vi "Complete Algorithm_Host.vi"() -> ()   [LabVIEW 2011]
uses:
  <vilib>/measure/NI_MAPro.lvlib
  <vilib>/Analysis/NI_AALBase.lvlib
  FFT/Controls/FFT States.ctl
  <vilib>/measure/maspectr.llb/FFT Spectrum (Mag-Phase) for 1 Chan (CDB).vi
  <vilib>/Analysis/1siggen.llb/Ramp Pattern by Samples.vi
  Interpolation Block/Controls/Interpolation Input Data.ctl
  <vilib>/Analysis/NI_AALPro.lvlib
  <vilib>/Analysis/2dsp.llb/Real FFT.vi
  <vilib>/gmath/NI_Gmath.lvlib
  FFT/Controls/FFT Parameters.ctl
panel:
  out "Resampled Waveform Error":dbl[](graph)=[-6.976252814558266, -5.323343553412211, -2.8114333153546744, -26.54772585626159, -19.783463943885028, -24.955368759801782, -31.021231527647238, -27.6461877092507, -38.95671779693381, -29.146757893293778, -40.920500463104865, -29.778667799092602, -30.651480033843615, -39.617647950762674, -29.777119057976908, -35.747085008088305, -35.2985019790654, -37.76767677188048, -33.9462465942451, -30.02327803942113, -39.37688378105776, -35.94385793381323, -35.585106057981605, -40.48040927607361, -32.74968635815885, -36.438287617816435, -47.755067442121316, -40.45338682146091, -52.23635514643328, -40.6295428448561, -38.1524909017659, -48.76110841180686, -40.71433935621975, -39.00688364486796, -56.49784789209585, -37.42986222843402, -40.49625037212847, -44.06886067307057, -38.31525964353108, -59.63457027143055, -35.566588313612634, -33.467351968403946, -36.68413625267246, -41.04536841104639, -42.31435254051097, -36.274070107607145, -37.150764121682805, -50.332950824589815, -46.20156369462504, -46.444900910375225, -44.8364219648814, -48.57917680413567, -42.19794262901505, -40.506737237586975, -52.63002253901345, -39.72758659866716, -38.214786945688516, -39.56035908067337, -43.32060173475149, -39.61076431387224, -33.093522184387204, -34.74046406069414, -45.152114353755366, -38.20642899575148, -42.09609113759559, -41.768976367924466, -38.66318028792905, -38.4756737843668, -39.924187998371096, -46.05349347381723, -35.49027459608772, -36.025415041989326, -38.51092517659433, -36.83569854602486, -40.795380624021725, -36.35991369515506, -37.81728427386544, -44.61046277229856, -35.266016721014964, -35.92322715684338, -42.88567587562287, -50.74251290714233, -44.872042376101916, -42.68123807149777, -42.92436430457484, -48.84492734632382, -45.3696804814589, -38.37702895182521, -40.36098970624832, -48.510609418962495, -57.25548500472812, -43.979468134992715, -38.14224729316644, -40.56618511041606, -58.13679214274917, -44.759022108404935, -40.256764450613, -41.685001222819444, -54.61994454936558, -44.38945314872701, -49.93473371978812, -46.25638908324654, -42.539518328159865, -45.28773309215987, -43.23721587175819, -45.564359245981514, -46.961044473626615, -41.32558704191926, -38.125744733097655]
  out "FFT_FXP_no DIT":dbl[](graph)=[-0.9553570049207104, 0.6968999494108972, 3.2074240707672486, -20.53122498149444, -13.77089446014236, -18.952463060127535, -25.022087351671377, -21.655924863873462, -32.972655817656346, -23.178155409959732, -34.96764173487915, -23.830599429203577, -24.72530525148686, -33.696009783345744, -23.883798703280526, -29.872860366292603, -29.438514987857264, -31.94494876745275, -28.134798131521784, -24.23918297363493, -33.63738541391448, -30.215293162386203, -29.890534838760058, -34.805342346114784, -27.123370304893385, -30.839734571250396, -42.17935864808424, -34.92729722281159, -46.65167705453899, -35.156781588661715, -32.71759437126826, -43.39065085727536, -35.35602088973465, -33.720145839352995, -51.22083266003117, -32.22975713342345, -35.372416231632016, -38.961220511182894, -33.295472896454925, -54.94205288567625, -30.643481005262174, -28.613588128886647, -31.89687360197505, -36.34212825746688, -37.630998520773005, -31.664986633794463, -32.60179747579538, -45.75845140392847, -41.84167849659361, -42.09857689345015, -40.617829297597325, -44.43194429667791, -38.11044261216089, -36.528827231710956, -48.782090563932016, -35.920982262632904, -34.50760172914073, -35.91963395980357, -39.7684802539758, -36.13416975134405, -29.703949311666285, -31.44846989771336, -41.95513728241616, -35.10351644257866, -39.07605566599686, -38.87160754828359, -35.91749374911157, -35.85331514008895, -37.44076426648204, -43.70958159602134, -33.21932185799169, -33.9061230773539, -36.55098574885896, -34.9837064659399, -39.08072335574801, -34.794348852725776, -36.39048296432991, -43.31555914578375, -34.19729522033075, -35.02592866181829, -42.21011656437949, -49.98820340744261, -44.37636412014499, -42.393601328796876, -42.88625468811113, -49.03715936994228, -45.71970468705827, -38.917038799967656, -41.10409295431466, -49.48714628994594, -58.85648271093962, -45.42701062252409, -39.84728347746511, -42.54601837493462, -60.621507019043705, -47.14439309014662, -42.94569780155637, -44.761084889164124, -57.83927091459509, -47.97668555883114, -54.11859137929727, -50.610961848127296, -47.29689223076528, -50.46072316096139, -48.986236804948476, -52.083879275586, -53.307091387367734, -48.16224363052139, -45.443188472860484, -45.23440881714418, -47.85854889637821, -56.27836973151929, -54.9658463374032, -52.46594288951086, -66.34887368032327, -55.304784228123715, -52.19923351123122, -49.138384495401304, -49.26606066713251, -57.96592937153396, -60.3194968415907, -55.628260569108406, -58.20499964743555, -68.60615252726132]
  in  "Resample Waveform Size":i32=1024
  out "Error 2":dbl[](graph)=[43.28680336773397, 54.874209998377815, 63.40667927216815, 43.19214378295915, 52.4550850459606, 49.22125785617935, 44.738870122314516, 49.45267259284084, 39.30177705005138, 50.134555753031705, 39.275704089007256, 51.245104293962626, 51.127749856906036, 42.85648338602506, 53.340338006756994, 47.96924132299105, 48.97797635960519, 47.034930612021746, 51.352355468446454, 55.7444416762564, 46.8358322946451, 50.69208531689444, 51.454318833795625, 46.94450536240401, 55.04425575816844, 51.709561920450575, 40.7327536810958, 48.36152013811606, 36.89368738030214, 48.80452194457727, 51.57523466078294, 41.25059427183906, 49.5722700549092, 51.54611873091486, 34.313540452847406, 53.63236777747285, 50.80970056229957, 47.47407920925422, 53.45829484965432, 32.363554263910956, 56.65036641185069, 58.962975235045974, 55.95436745637467, 51.796359091271164, 50.72587252279395, 56.960137493066384, 56.273108272838066, 43.27645317017654, 47.589411598739304, 47.523847575579595, 49.30645397147554, 45.73432415131559, 52.282815875412304, 54.1380385934558, 42.17565050739418, 55.23597705017646, 56.90376805485219, 55.710389681351565, 52.09963955408854, 55.95635968044763, 62.61796149748388, 61.11293878909635, 50.84084561754173, 57.92380075640719, 54.169192230434234, 54.62921231546552, 57.86583016583704, 58.182136728381984, 56.860459946783195, 50.856085773727784, 61.54238388111302, 61.128522348534126, 58.762540395168074, 60.55559200683594, 56.71207730112699, 61.262097748384264, 59.91770884995849, 53.235980561308736, 62.69038415636078, 62.141675919302926, 55.28630996648335, 47.535170841473615, 53.509987719815285, 55.80381890136056, 55.66243101034867, 49.84234761250371, 53.41684421245931, 60.50754335878166, 58.620454939783315, 50.56655820817769, 41.916281306637835, 55.28579679006381, 61.21543960663583, 58.88286979638478, 41.40259874663488, 54.869693985418834, 59.46028664791151, 58.11941461888414, 45.27088509828608, 55.5868581029331, 50.12614510390771, 53.88816090765136, 57.68782353080626, 55.02153794034635, 57.15313776263364, 54.906246078218906, 53.58899684214845, 59.30308935204265, 62.58078019747132]
  out "Resampled Waveform FXP":dbl[](graph)=[-6.976252814558266, -5.323343553412211, -2.8114333153546744, -26.54772585626159, -19.783463943885028, -24.955368759801782, -31.021231527647238, -27.6461877092507, -38.95671779693381, -29.146757893293778, -40.920500463104865, -29.778667799092602, -30.651480033843615, -39.617647950762674, -29.777119057976908, -35.747085008088305, -35.2985019790654, -37.76767677188048, -33.9462465942451, -30.02327803942113, -39.37688378105776, -35.94385793381323, -35.585106057981605, -40.48040927607361, -32.74968635815885, -36.438287617816435, -47.755067442121316, -40.45338682146091, -52.23635514643328, -40.6295428448561, -38.1524909017659, -48.76110841180686, -40.71433935621975, -39.00688364486796, -56.49784789209585, -37.42986222843402, -40.49625037212847, -44.06886067307057, -38.31525964353108, -59.63457027143055, -35.566588313612634, -33.467351968403946, -36.68413625267246, -41.04536841104639, -42.31435254051097, -36.274070107607145, -37.150764121682805, -50.332950824589815, -46.20156369462504, -46.444900910375225, -44.8364219648814, -48.57917680413567, -42.19794262901505, -40.506737237586975, -52.63002253901345, -39.72758659866716, -38.214786945688516, -39.56035908067337, -43.32060173475149, -39.61076431387224, -33.093522184387204, -34.74046406069414, -45.152114353755366, -38.20642899575148, -42.09609113759559, -41.768976367924466, -38.66318028792905, -38.4756737843668, -39.924187998371096, -46.05349347381723, -35.49027459608772, -36.025415041989326, -38.51092517659433, -36.83569854602486, -40.795380624021725, -36.35991369515506, -37.81728427386544, -44.61046277229856, -35.266016721014964, -35.92322715684338, -42.88567587562287, -50.74251290714233, -44.872042376101916, -42.68123807149777, -42.92436430457484, -48.84492734632382, -45.3696804814589, -38.37702895182521, -40.36098970624832, -48.510609418962495, -57.25548500472812, -43.979468134992715, -38.14224729316644, -40.56618511041606, -58.13679214274917, -44.759022108404935, -40.256764450613, -41.685001222819444, -54.61994454936558, -44.38945314872701, -49.93473371978812, -46.25638908324654, -42.539518328159865, -45.28773309215987, -43.23721587175819, -45.564359245981514, -46.961044473626615, -41.32558704191926, -38.125744733097655]
  in  "other option":fxp<+,10,10>=362.0 format="%.0b"
  out "Error":dbl[](graph)=[49.30769917737152, 60.89445350120092, 69.42553665829007, 49.2086446577263, 58.46765452970327, 55.2241635558536, 50.73801429829038, 55.44293543821807, 45.28583902932884, 56.10315823636576, 45.22856281723297, 57.193172663851655, 57.05392463926279, 48.77812155344199, 59.23365836145337, 53.84346596478676, 54.837963350813325, 52.85765861644948, 57.163803931169774, 61.528536742042604, 52.57533066178838, 56.420650088321466, 57.14889005301717, 52.61957229236283, 60.6705718114339, 57.308114967016614, 46.30846247513288, 53.887609736765384, 42.47836547219643, 54.27728320077165, 57.01013119128058, 46.62105182637056, 54.9305885213943, 56.83285653642983, 39.59055568491208, 58.83247287248342, 55.933534702796024, 52.581719371141894, 58.478081596730476, 37.056071649665256, 61.57347372020115, 63.81673907456327, 60.74163010707208, 56.49959924485067, 55.40922654253191, 61.569220966879065, 60.82207491872549, 47.850952590837885, 51.94929679677073, 51.87017159250467, 53.52504663875962, 49.88155665877335, 56.37031589226647, 58.11594859933182, 46.02358248247562, 59.04258138621071, 60.61095327139998, 59.35111480222137, 55.65176103486423, 59.432954242975825, 66.00753437020481, 64.40493295207713, 54.03782268888094, 61.02671330958001, 57.189227702032966, 57.5265811351064, 60.61151670465452, 60.80449537265983, 59.34388367867225, 53.199997651523674, 63.81333661920905, 63.247814313169556, 60.72247982290344, 62.40758408692089, 58.4267345694007, 62.827662590813546, 61.344510159494014, 54.530884187823546, 63.75910565704499, 63.03897441432802, 55.961869277726734, 48.28948034117333, 54.00566597577221, 56.091455644061455, 55.700540626812376, 49.65011558888525, 53.06682000685994, 59.967533510639214, 57.877351691716974, 49.590021337194244, 40.31528360042633, 53.83825430253244, 59.51040342233716, 56.90303653186622, 38.91788387034035, 52.48432300367715, 56.77135329696814, 55.04333095253946, 42.05155873305657, 51.999625692828964, 45.94228744439856, 49.533588142770604, 52.93044962820085, 49.848547871544824, 51.40411682944335, 48.38672604861442, 47.24294992840733, 52.46643276344052, 55.26333645770849, 55.54919208244534, 53.00136899535208, 44.65711939676295, 46.04448113696606, 48.61850256209727, 34.80898156988724, 45.925784512432905, 49.10336397303664, 52.23556824940267, 52.17858483047705, 43.548757068298144, 41.26458915804296, 46.02459377600748, 43.51600174544239, 33.18238428896369]
  out "Iterations":i32=1309
  in  "Intersperse Ratio":dbl=0.1
  in  "Stimulus Type":enum16{"Sine", "Ramp", "Chirp"}(ring)
  in  "Samples":i32=1600
  out "Test Progress (%)":dbl(slide)=99.92360580595874 scale=0.0..100.0
  out "Error Signal":dbl[](graph)=[43.27868118229223, 54.86552230179002, 63.389987587522825, 43.18908838922074, 52.449486489845626, 49.211782865981135, 44.732757899961754, 49.44651655209154, 39.28974484698519, 50.132876146325486, 39.27042330211212, 51.23080334305523, 51.12688614074965, 42.856943836787735, 53.3244883147339, 47.96632633107936, 48.967884588670586, 47.02526363390223, 51.34547706269156, 55.73256346567753, 46.83380982570286, 50.67891200070767, 51.44176864177723, 46.93663338847762, 55.04003586632729, 51.70644328826701, 40.72610237321712, 48.35006320957697, 36.89176127673542, 48.793439789433364, 51.56366306254884, 41.24607768364592, 49.56004691112895, 51.537377375782825, 34.30357584494325, 53.63254250590687, 50.80595093442804, 47.46481488232479, 53.4571482431854, 32.3653120353415, 56.650548475463324, 58.95376470344992, 55.95490995904713, 51.78704000231755, 50.723818813304916, 56.95686385067353, 56.27152864452087, 43.26565399476635, 47.58394404336434, 47.51952973595482, 49.299125936356944, 45.73146970545126, 52.27763350442736, 54.13305708104278, 42.172860546407634, 55.22918864884362, 56.89980500054071, 55.70824876202494, 52.09602253884003, 55.94993649431987, 62.61382743187109, 61.111215349790484, 50.8367099712971, 57.91147975215867, 54.15590836802983, 54.62865743338999, 57.86104170376609, 58.16952926274878, 56.85105419515429, 50.85489174754501, 61.54047097720074, 61.11487489052345, 58.7539343217624, 60.551446802860795, 56.710582925148714, 61.25482394353932, 59.91077437382393, 53.2331620836073, 62.67905712737574, 62.13912182614631, 55.281360842106224, 47.52377749861594, 53.5070300959172, 55.80146322285833, 55.653201564923506, 49.83571245882753, 53.41543094391821, 60.49785356060687, 58.61035089603163, 50.557636377140184, 41.91786006136596, 55.28088992505653]
  out "LabVIEW FFT":dbl[](graph)=[-50.26305618229223, -60.19755355179002, -66.21811258752282, -69.73986963922074, -72.23854898984563, -74.17662661598114, -75.76010164996175, -77.09886030209154, -78.25849484698519, -79.28131364632549, -80.19620455211212, -81.02377209305523, -81.77922989074965, -82.47413133678774, -83.1174570647339, -83.71632633107936, -84.27647833867059, -84.80260738390223, -85.29860206269156, -85.76771971567753, -86.21271607570286, -86.63594325070767, -87.03942489177723, -87.42491463847762, -87.79394211632729, -88.14784953826701, -88.48782112321712, -88.81490695957697, -89.13004252673542, -89.43406478943336, -89.72772556254884, -90.01170268364592, -90.28660941112895, -90.55300237578282, -90.81138834494325, -91.06223000590687, -91.30595093442804, -91.54293988232479, -91.7735544931854, -91.9981245353415, -92.21695472546332, -92.43032720344992, -92.63850370904713, -92.84172750231755, -93.04022506330492, -93.23420760067353, -93.42387239452087, -93.60940399476635, -93.79097529336434, -93.96874848595482, -94.14287593635694, -94.31350095545126, -94.48075850442736, -94.64477583104278, -94.80567304640763, -94.96356364884362, -95.11855500054071, -95.27074876202494, -95.42024128884003, -95.56712399431987, -95.71148368187109, -95.85340284979048, -95.9929599712971, -96.13022975215867, -96.26528336802983, -96.39818868338999, -96.52901045376609, -96.65781051274878, -96.78464794515429, -96.90957924754501, -97.03265847720074, -97.15393739052345, -97.2734655717624, -97.3912905528608, -97.50745792514871, -97.62201144353932, -97.73499312382393, -97.8464433336073, -97.95640087737574, -98.06490307614631, -98.17198584210622, -98.27768374861594, -98.3820300959172, -98.48505697285833, -98.5867953149235, -98.68727495882753, -98.78652469391821, -98.88457231060687, -98.98144464603163, -99.07716762714018, -99.17176631136596, -99.26526492505653, -99.35768689980227, -99.44905490680084, -99.53939088938405, -99.62871609382377, -99.71705109852451, -99.80441584170359, -99.89082964765166, -99.9763112516601, -100.06087882369583, -100.1445499908979, -100.22734185896613, -100.30927103250622, -100.39035363439183, -100.47060532420042, -100.55004131577506, -100.62867639396191, -100.70652493056897, -100.78360089958952, -100.85991789173029, -100.93548912828224, -101.01032747436926, -101.08444545160813, -101.1578552502105, -101.23056874055662, -101.30259748426786, -101.37395274480397, -101.44464549760956, -101.5146864398321, -101.58408599963366, -101.65285434511588, -101.72100139287794, -101.788536816225, -101.85547005304441, -101.92181031336544, -101.98756658661802, -102.05274764860431, -102.11736206819708, -102.18141821377729, -102.24492425942302, -102.3078881908616, -102.37031781119495, -102.4322207464091, -102.49360445067742, -102.55447621146658, -102.61484315445394, -102.67471224826505, -102.73409030903872, -102.79298400482733, -102.85139985983925, -102.90934425853058, -102.9668234495519, -103.02384354955689, -103.08041054687794, -103.13653030507479, -103.19220856636092, -103.24745095491336, -103.30226298007, -103.35665003941926, -103.41061742178658, -103.46417031012149, -103.51731378428946, -103.57005282377227, -103.62239231028016, -103.6743370302799, -103.72589167744084, -103.77706085500365, -103.82784907807306, -103.87826077583887, -103.92830029372675, -103.97797189548271, -104.02727976519243, -104.07622800923858, -104.12482065819847, -104.17306166868394, -104.22095492512537, -104.26850424150248, -104.31571336302333, -104.36258596775329, -104.40912566819617, -104.45533601282891, -104.50122048759147, -104.54678251733358, -104.5920254672197, -104.63695264409375, -104.68156729780503, -104.72587262249638, -104.76987175785621, -104.81356779033534, -104.85696375433007, -104.90006263333213, -104.94286736104739, -104.98538082248362, -105.02760585500863, -105.0695452493797, -105.11120175074538, -105.15257805962035, -105.19367683283409, -105.23450068445472, -105.2750521866882, -105.31533387075385, -105.35534822773724, -105.39509770942082, -105.4345847290931, -105.47381166233664, -105.51278084779648, -105.55149458792862, -105.58995514972962, -105.62816476544788, -105.6661256332768, -105.7038399180312, -105.74130975180621, -105.77853723462044, -105.81552443504323, -105.85227339080623, -105.88878610940054, -105.925064568659, -105.96111071732466, -105.9969264756055, -106.03251373571594, -106.06787436240538, -106.10301019347443, -106.13792304027876, -106.17261468822122, -106.2070868972325, -106.24134140224058, -106.27537991362941, -106.30920411768679, -106.34281567704234, -106.37621623109517, -106.40940739643204, -106.4423907672358, -106.47516791568513, -106.50774039234466, -106.54010972654694, -106.57227742676562, -106.60424498098058, -106.63601385703471, -106.66758550298329, -106.69896134743531, -106.73014279988772, -106.76113125105216, -106.79192807317493, -106.8225346203498, -106.85295222882439, -106.88318221729975, -106.91322588722397, -106.9430845230792, -106.97275939266288, -107.002251747363, -107.03156282242757, -107.0606938372286, -107.08964599552061, -107.11842048569372, -107.14701848102146, -107.17544113990401, -107.2036896061057, -107.23176500898845, -107.25966846374018, -107.28740107159814, -107.31496392006888, -107.3423580831428, -107.36958462150467, -107.39664458274078, -107.4235390015406, -107.45026889989595, -107.47683528729388, -107.50323916091043, -107.52948150579486, -107.55556329505436, -107.58148549003349, -107.60724904049107, -107.63285488477297, -107.65830394998153, -107.6835971521424, -107.70873539636813, -107.73371957701785, -107.75855057785493, -107.78322927220125, -107.80775652308833, -107.83213318340628, -107.85636009604951, -107.88043809405976, -107.90436800076678, -107.92815062992617, -107.95178678585475, -107.97527726356363, -107.99862284888852, -108.02182431861806, -108.04488244061963, -108.06779797396277, -108.09057166904077, -108.11320426768967, -108.13569650330543, -108.15804910095886, -108.18026277750859, -108.20233824171198, -108.22427619433424, -108.24607732825534, -108.26774232857547, -108.2892718727181, -108.31066663053198, -108.33192726439057, -108.35305442929038, -108.37404877294733, -108.39491093589157, -108.41564155156043, -108.43624124639022, -108.45671063990613, -108.47705034481058, -108.49726096707036, -108.51734310600206, -108.53729735435616, -108.55712429839967, -108.57682451799745, -108.59639858669206, -108.61584707178247, -108.63517053440123, -108.65436952959053, -108.67344460637702, -108.69239630784531, -108.7112251712102, -108.72993172788797, -108.74851650356632, -108.76698001827322, -108.78532278644448, -108.80354531699071, -108.8216481133626, -108.8396316736155, -108.85749649047293, -108.87524305138903, -108.89287183860998, -108.91038332923442, -108.92777799527309, -108.94505630370729, -108.96221871654659, -108.97926569088547, -108.99619767895926, -109.01301512819904, -109.02971848128578, -109.0463081762035, -109.06278464629175, -109.0791483202973, -109.09539962242475, -109.11153897238664, -109.12756678545279, -109.14348347249854, -109.1592894400527, -109.17498509034445, -109.19057082134958, -109.20604702683616, -109.22141409640923, -109.23667241555522, -109.25182236568524, -109.26686432417804, -109.28179866442221, -109.29662575585766, -109.3113459640166, -109.32595965056382, -109.34046717333646, -109.35486888638302, -109.36916514000201, -109.3833562807796, -109.39744265162722, -109.41142459181849, -109.42530243702515, -109.43907651935297, -109.45274716737686, -109.46631470617562, -109.47977945736604, -109.49314173913638, -109.5064018662798, -109.5195601502268, -109.53261689907737, -109.54557241763283, -109.5584270074269, -109.57118096675649, -109.58383459071209, -109.5963881712075, -109.60884199700935, -109.62119635376601, -109.63345152403616, -109.645607787317, -109.65766542007185, -109.66962469575755, -109.68148588485137, -109.69324925487756, -109.70491507043334, -109.71648359321486, -109.72795508204234, -109.73932979288529, -109.75060797888703, -109.76178989038894, -109.77287577495434, -109.78386587739226, -109.79476043978053, -109.80555970148855, -109.8162638991999, -109.82687326693474, -109.83738803607153, -109.84780843536852, -109.85813469098514, -109.86836702650291, -109.87850566294597, -109.88855081880166, -109.89850271004013, -109.90836155013452, -109.91812755008, -109.92780091841328, -109.93738186123122, -109.9468705822094, -109.95626728262069, -109.96557216135307, -109.97478541492741, -109.98390723751511, -109.99293782095518, -110.0018773547713, -110.01072602618864, -110.01948402015012, -110.0281515193329, -110.03672870416412, -110.04521575283678, -110.05361284132533, -110.06192014340064, -110.07013783064536, -110.07826607246854, -110.0863050361202, -110.09425488670585, -110.10211578720038, -110.10988789846218, -110.11757137924667, -110.12516638621992, -110.13267307397183, -110.1400915950292, -110.14742209986862, -110.15466473692908, -110.16181965262444, -110.16888699135563, -110.17586689552282, -110.18275950553712, -110.18956495983231, -110.19628339487633, -110.20291494518258, -110.20945974332093, -110.21591791992869, -110.22228960372134, -110.22857492150307, -110.23477399817709, -110.24088695675593, -110.24691391837136, -110.25285500228424, -110.25871032589433, -110.26448000474954, -110.27016415255545, -110.2757628811845, -110.28127630068465, -110.28670451928886, -110.29204764342307, -110.29730577771515, -110.3024790250031, -110.3075674863432, -110.31257126101838, -110.31749044654549, -110.32232513868362, -110.32707543144139, -110.33174141708434, -110.33632318614251, -110.34082082741716, -110.34523442798809, -110.34956407322026, -110.35380984677067, -110.35797183059466, -110.36205010495263, -110.36604474841597, -110.3699558378735, -110.37378344853721, -110.37752765394825, -110.38118852598252, -110.38476613485645, -110.38826054913221, -110.39167183572306, -110.3950000598987, -110.39824528529005, -110.40140757389432, -110.40448698607976, -110.40748358059018, -110.41039741454966, -110.41322854346683, -110.41597702123907, -110.4186429001567, -110.42122623090702, -110.42372706257805, -110.4261454426625, -110.42848141706114, -110.43073503008645, -110.43290632446605, -110.43499534134575, -110.43700212029285, -110.43892669929905, -110.44076911478349, -110.44252940159527, -110.44420759301629, -110.44580372076373, -110.4473178149923, -110.44874990429682, -110.45010001571418, -110.45136817472532, -110.4525544052573, -110.4536587296852, -110.45468116883347, -110.45562174197784, -110.45648046684661, -110.45725735962185, -110.45795243494119, -110.45856570589812, -110.45909718404366, -110.45954687938678, -110.45991480039524, -110.46020095399682, -110.46040534557864, -110.46052797898855]
  out "LabVIEW Input":dbl[](graph)=[-0.9553570049207104, 0.6968999494108972, 3.2074240707672486, -20.53122498149444, -13.77089446014236, -18.952463060127535, -25.022087351671377, -21.655924863873462, -32.972655817656346, -23.178155409959732, -34.96764173487915, -23.830599429203577, -24.72530525148686, -33.696009783345744, -23.883798703280526, -29.872860366292603, -29.438514987857264, -31.94494876745275, -28.134798131521784, -24.23918297363493, -33.63738541391448, -30.215293162386203, -29.890534838760058, -34.805342346114784, -27.123370304893385, -30.839734571250396, -42.17935864808424, -34.92729722281159, -46.65167705453899, -35.156781588661715, -32.71759437126826, -43.39065085727536, -35.35602088973465, -33.720145839352995, -51.22083266003117, -32.22975713342345, -35.372416231632016, -38.961220511182894, -33.295472896454925, -54.94205288567625, -30.643481005262174, -28.613588128886647, -31.89687360197505, -36.34212825746688, -37.630998520773005, -31.664986633794463, -32.60179747579538, -45.75845140392847, -41.84167849659361, -42.09857689345015, -40.617829297597325, -44.43194429667791, -38.11044261216089, -36.528827231710956, -48.782090563932016, -35.920982262632904, -34.50760172914073, -35.91963395980357, -39.7684802539758, -36.13416975134405, -29.703949311666285, -31.44846989771336, -41.95513728241616, -35.10351644257866, -39.07605566599686, -38.87160754828359, -35.91749374911157, -35.85331514008895, -37.44076426648204, -43.70958159602134, -33.21932185799169, -33.9061230773539, -36.55098574885896, -34.9837064659399, -39.08072335574801, -34.794348852725776, -36.39048296432991, -43.31555914578375, -34.19729522033075, -35.02592866181829, -42.21011656437949, -49.98820340744261, -44.37636412014499, -42.393601328796876, -42.88625468811113, -49.03715936994228, -45.71970468705827, -38.917038799967656, -41.10409295431466, -49.48714628994594, -58.85648271093962, -45.42701062252409, -39.84728347746511, -42.54601837493462, -60.621507019043705, -47.14439309014662, -42.94569780155637, -44.761084889164124, -57.83927091459509, -47.97668555883114, -54.11859137929727, -50.610961848127296, -47.29689223076528, -50.46072316096139, -48.986236804948476, -52.083879275586, -53.307091387367734, -48.16224363052139, -45.443188472860484, -45.23440881714418, -47.85854889637821, -56.27836973151929, -54.9658463374032, -52.46594288951086, -66.34887368032327, -55.304784228123715, -52.19923351123122, -49.138384495401304, -49.26606066713251, -57.96592937153396, -60.3194968415907, -55.628260569108406, -58.20499964743555, -68.60615252726132]
  out "Error Spectrum":cluster{"f0":dbl, "df":dbl, "magnitude":dbl[]}(graph)={"f0"=-0.5, "df"=0.010869565217391304, "magnitude"=[-32.440172876894145, -15.649094048721865, -4.45919906126372, -1.0934248518747132, -3.5749189132785144, -13.856285825512536, -10.851361901545019, -7.260946617939843, -4.181045998412335, 0.6275260150758217, 3.6048161620768697, 1.223354659799965, 1.1089262180204518, 0.9163643256160556, 0.6465693287426431, -7.483194351185092, -14.142227893339083, -23.424392136210766, -11.528050727904443, -4.198774040275538, -5.551065197044159, -0.27154770951318674, 2.459716303433924, -1.1377109714444595, -2.1008637945935624, -5.036691738347846, -2.0215022938521625, 0.0733119225332626, 0.7054386897333763, -2.2298466343743026, -5.414052150634547, -3.94343537736747, -13.978340482907793, -8.845925214778124, -11.920377443982415, -9.493633116880673, -5.175332438602855, -5.841828513906063, -5.341665176637246, -2.8456561246200125, -0.839482446341243, 1.9228139979641963, 0.584568286382059, -4.8476893542846415, 0.7157070074941217, 28.10847166375863, 34.25230511529585, 28.10847166375863, 0.7157070074941217, -4.847689354284642, 0.5845682863820572, 1.9228139979641976, -0.8394824463412419, -2.845656124620011, -5.341665176637246, -5.841828513906058, -5.1753324386028465, -9.49363311688067, -11.920377443982431, -8.845925214778134, -13.978340482907807, -3.94343537736747, -5.414052150634545, -2.2298466343743013, 0.7054386897333763, 0.0733119225332626, -2.0215022938521625, -5.036691738347847, -2.100863794593554, -1.1377109714444595, 2.459716303433914, -0.27154770951318974, -5.551065197044165, -4.1987740402755405, -11.528050727904445, -23.42439213621077, -14.14222789333908, -7.483194351185097, 0.6465693287426394, 0.9163643256160537, 1.1089262180204484, 1.2233546597999632, 3.6048161620768715, 0.6275260150758217, -4.181045998412335, -7.260946617939843, -10.851361901545015, -13.856285825512533, -3.5749189132785144, -1.093424851874714, -4.45919906126372, -15.64909404872174]}
  out "FFT Overflow?":bool
  in  "FFT Parameters":T1={"Direction"=TRUE, "scale_sch"=362.0, "Flush Length"=1500} {"scale_sch" format="%.0b"}
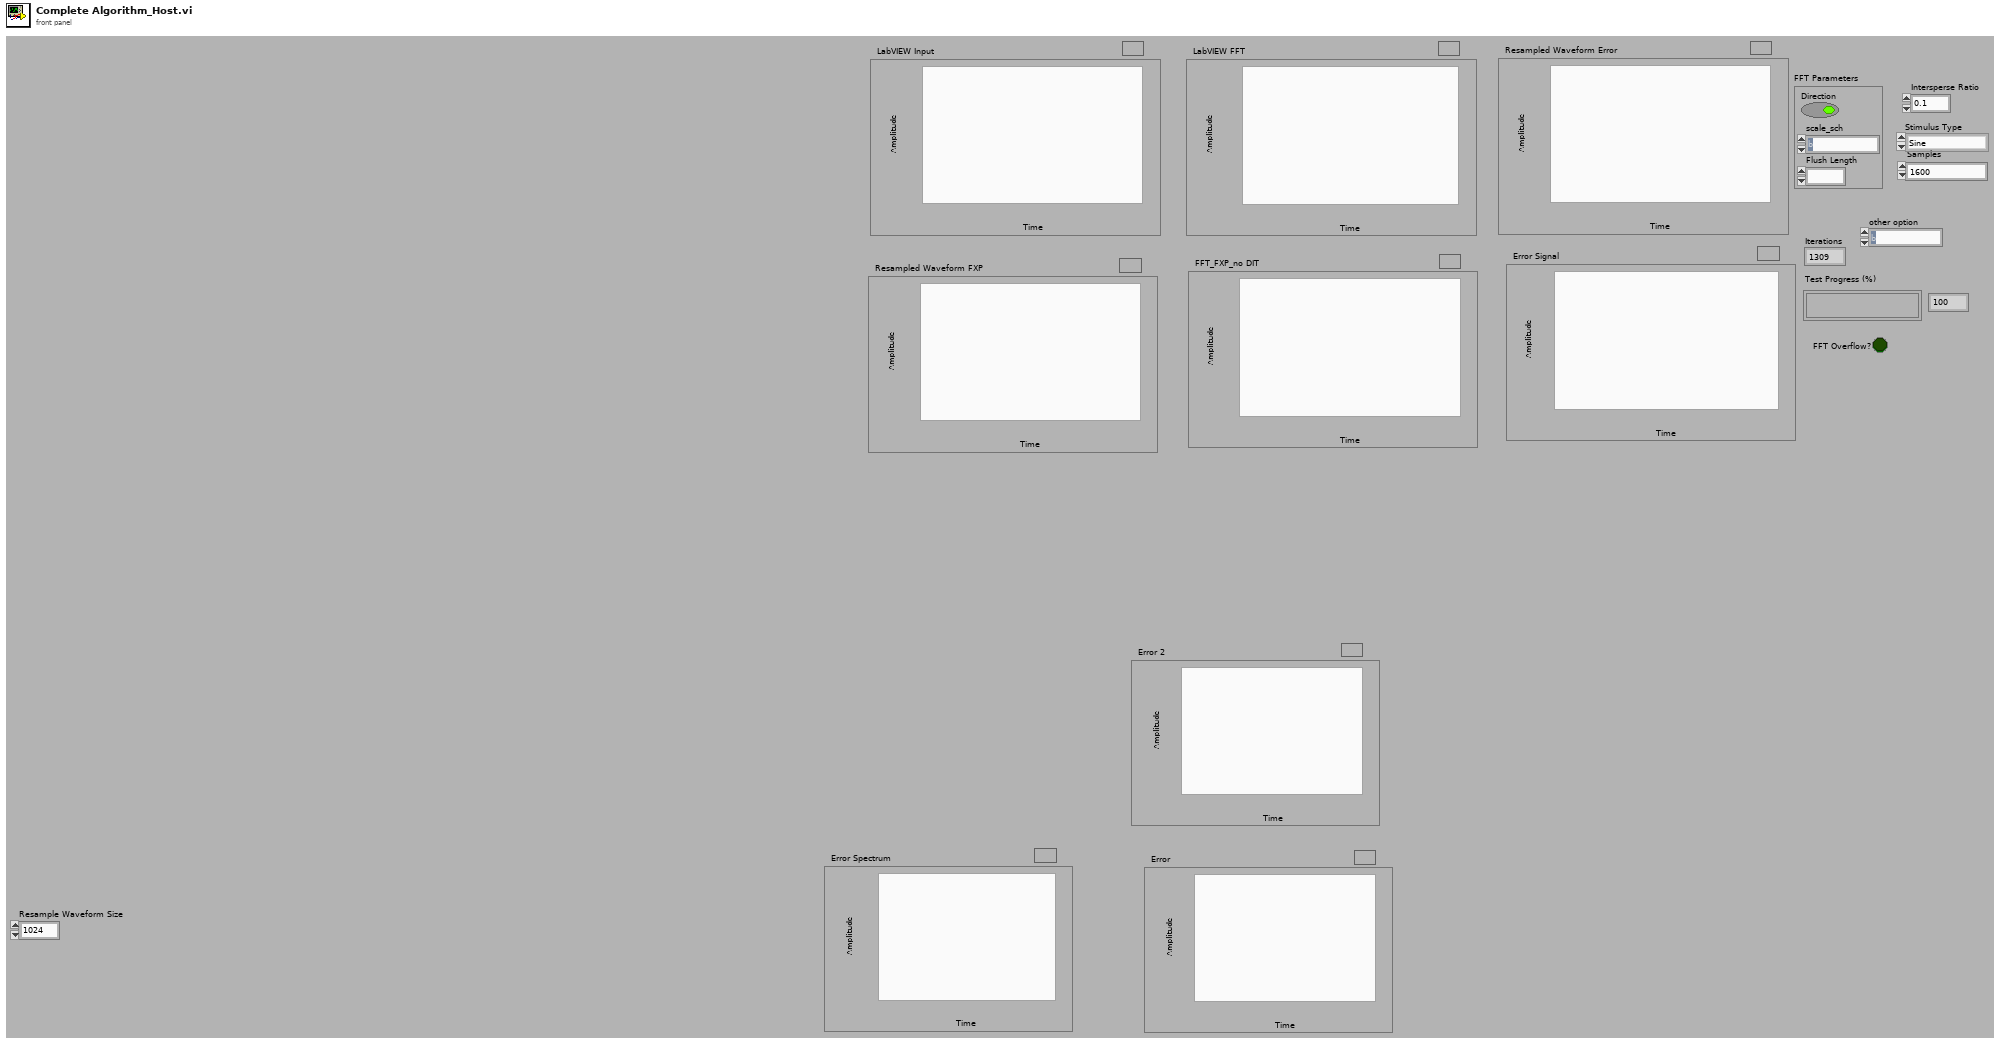
[diagram p1: front panel]
types:
  T1 = typedef "FFT Parameters.ctl" = cluster{"Direction":bool, "scale_sch":fxp<+,10,10>, "Flush Length":u16}
  T2 = typedef "FFT States.ctl" = enum8{"Configure", "Start FFT processing", "Process", "Unload Last FFT", "Reset"}
  T3 = cluster{"dB On (F)":bool, "unwrap phase (F)":bool, "convert to degree (F)":bool}
  T4 = typedef "Interpolation Input Data.ctl" = fxp<+/-,18,1>
  T5 = typedef "Interpolation Output Data.ctl" = fxp<+/-,19,1>
  T6 = cluster{"edone":bool, "FFT Overflow":bool, "Input Index":fxp<+,9,9>}
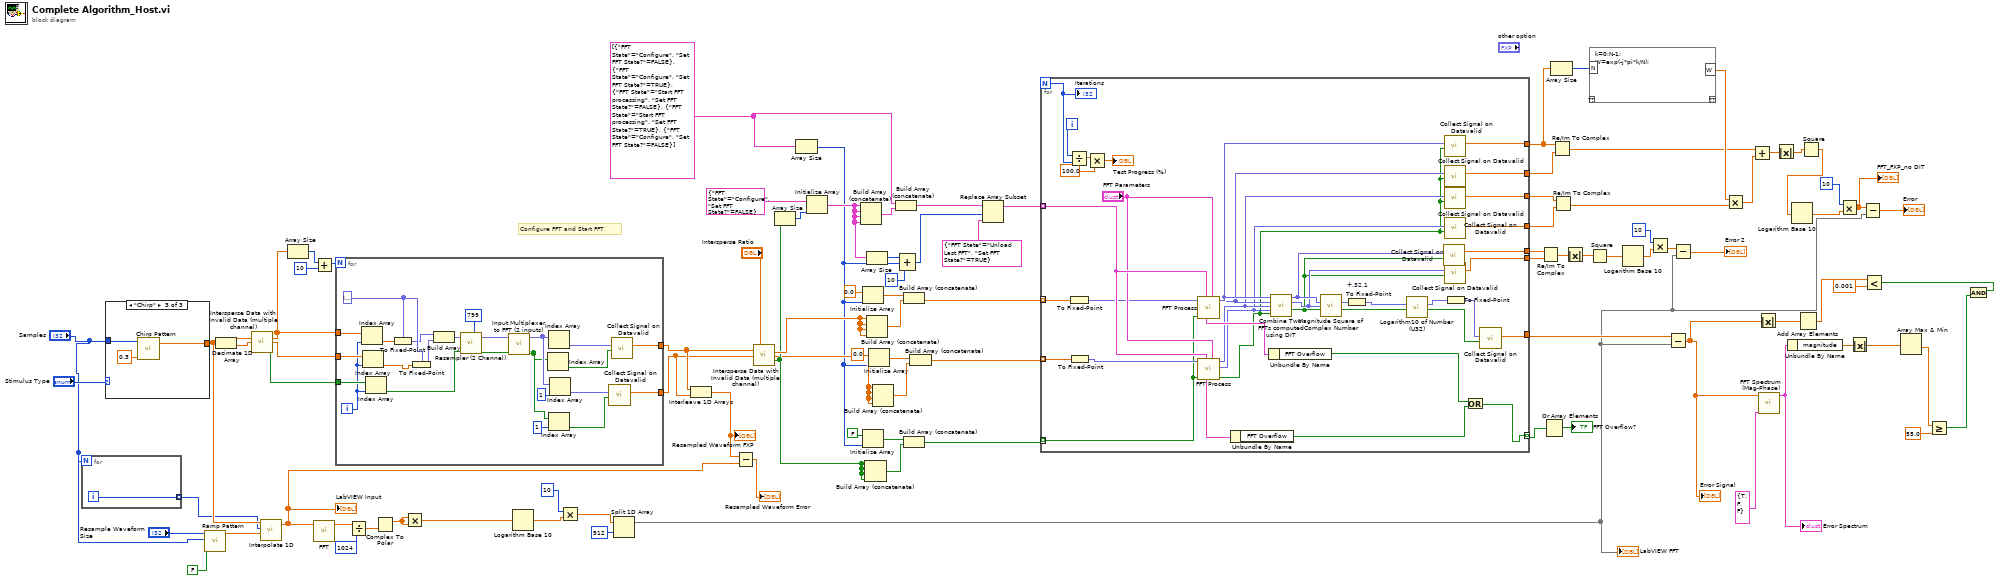
[diagram p0: block diagram]
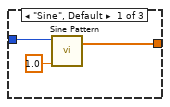
[diagram p2: hidden frame]
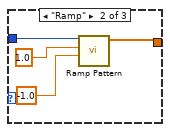
[diagram p3: hidden frame]
diagram:
  w73 = cluster{"FFT State":T2, "Set FFT State?":bool}[] [{"FFT State"=enum."Configure", "Set FFT State?"=FALSE}, {"FFT State"=enum."Configure", "Set FFT State?"=TRUE}, {"FFT State"=enum."Start FFT processing", "Set FFT State?"=FALSE}, {"FFT State"=enum."Start FFT processing", "Set FFT State?"=TRUE}, {"FFT State"=enum."Configure", "Set FFT State?"=FALSE}]
  # "Configure FFT and Start FFT"
  n1 = for {
    N: "Samples" -> [_]
    tunnel: [w99] -> w8 mode=indexing
    i -> [w99]
  }
  n2 = case shown="\"Chirp\"" "Stimulus Type" {
    tunnel: "Samples" -> [w102 w104 w109]
    tunnel: [w100 w103 w108] -> w14
    frame "Sine", Default {
      n3 = call <vilib>:"Sine Pattern.vi"("cycles"=1.0, "samples"=w102) -> ("Sinusoidal Pattern"=w100:dbl[])  [unwired: 2 in, 1 out]
    }
    frame "Ramp" {
      n4 = call-poly <vilib>:"Ramp Pattern.vi"("start"=-1.0, "end"=1.0, "samples"=w104) -> ("Ramp Pattern"=w103:dbl[])  [unwired: 7 in, 1 out]
    }
    frame "Chirp" {
      n5 = call <vilib>:"Chirp Pattern.vi"("f2"=0.3, "samples"=w109) -> ("Chirp Pattern"=w108:dbl[])  [unwired: 2 in, 1 out]
    }
  }
  n6 = call-poly <vilib>:"Ramp Pattern.vi"("exclude end?"=FALSE, "end"="Samples", "samples"="Resample Waveform Size") -> ("Ramp Pattern"=w15:dbl[])  [unwired: 7 in, 1 out]
  n7 = Decimate 1D Array(w14) -> (w26:dbl[], w29:dbl[])
  n8 = call <userlib>:"Intersperse Data with Invalid Data (multiple channel).vi"("Channel0 Input"=w26, "Channel1 Input"=w29) -> ("Channel0 Output"=w2:dbl[], "Channel1 Output"=w28:dbl[], "Data Valid"=w27:bool[])  [unwired: 11 in]
  n9 = call <vilib>:"Interpolate 1D.vi"("xi"=w15, "X"=w8, "Y"=w14) -> ("yi"=w4:dbl[])  [unwired: 6 in, 2 out]
  "LabVIEW Input" <- w4
  n10 = Array Size(array=w2) -> (size(s)=w25:i32)
  n11 = call-poly <vilib>:"FFT.vi"("X"=w4) -> ("FFT {X}"=w21:cdb[])  [unwired: 9 in, 1 out]
  n12 = Add(x=w25, y=10) -> (x+y=w23:i32)
  n13 = for {
    N: w23 -> [_]
    tunnel: w2 -> [w132]
    tunnel: w28 -> [w131]
    tunnel: w27 -> [w130]
    tunnel: [w118] -> w10
    tunnel: [w117] -> w9
    i -> [w128]
    w125 = T4 0.0 ("Interpolate.Input Data")
    n14 = Index Array(array=w132, index=w128) -> (element=w127:dbl)
    n15 = Index Array(array=w131, index=w128) -> (element=w126:dbl)
    n16 = Index Array(array=w130, index=w128) -> (element=w129:bool)
    n17 = To Fixed-Point(fixed-point type=w125, number=w127) -> (fixed-point=w123:T4)
    n18 = To Fixed-Point(fixed-point type=w125, number=w126) -> (fixed-point=w124:T4)
    n19 = Build Array(w123, w124) -> (w122:T4[])
    n20 = call "Resampler (2 Channel).vi"("CalibrationTable Length-1"=u16 799 ("Table Length-1"), "DataValid"=w129, "Input Data"=w122) -> ("Data Valid"=w120:bool[], "Interpolated Data"=w121:T5[])  [unwired: 7 in]
    n21 = call "Input Multiplexer to FFT (2 inputs).vi"("Input Data Valid Array"=w120, "Input Data"=w121) -> ("Output Data Valid Array"=w114:bool[], "Interchanged Data"=w115:T5[])  [unwired: 8 in]
    n22 = Index Array(array=w114) -> (element=w116:bool)  [unwired: 1 in]
    n23 = Index Array(array=w115) -> (element=w119:T5)  [unwired: 1 in]
    n24 = Index Array(array=w114, index=1) -> (element=w111:bool)
    n25 = Index Array(array=w115, index=1) -> (element=w110:T5)
    n26 = call <userlib>:"Collect Signal on Datavalid.vi"("Data Valid"=w111, "Input"=w110) -> ("Output"=w117:dbl[])  [unwired: 9 in]
    n27 = call <userlib>:"Collect Signal on Datavalid.vi"("Data Valid"=w116, "Input"=w119) -> ("Output"=w118:dbl[])  [unwired: 9 in]
  }
  n28 = Divide(x=w21, y=1024) -> (x/y=w19:cdb[])
  n29 = Complex To Polar(r * e^(i*theta)=w19) -> (r=w18:dbl[])  [unwired: 1 out]
  n30 = Multiply(x=w18, y=w18) -> (x*y=w17:dbl[])
  n31 = Logarithm Base 10(1:w17) -> (0:w22:dbl[])
  n32 = Multiply(x=10, y=w22) -> (x*y=w12:dbl[])
  n33 = Split 1D Array(array=w12, index=512) -> (first subarray=w11:dbl[])  [unwired: 1 out]
  "LabVIEW FFT" <- w11
  n34 = Interleave 1D Arrays(w10, w9) -> (w5:dbl[])
  "Resampled Waveform FXP" <- w5
  n35 = Subtract(x=w5, y=w4) -> (x-y=→"Resampled Waveform Error":dbl[])
  n36 = call <userlib>:"Intersperse Data with Invalid Data (multiple channel).vi"("Intersperse Ratio"="Intersperse Ratio", "Channel0 Input"=w10, "Channel1 Input"=w9) -> ("Channel0 Output"=w66:dbl[], "Channel1 Output"=w58:dbl[], "Data Valid"=w64:bool[])  [unwired: 10 in]
  n37 = Array Size(array=w64) -> (size(s)=w65:i32)
  n38 = Array Size(array=w73) -> (size(s)=w57:i32)
  n39 = Initialize Array(cluster{"FFT State":T2, "Set FFT State?":bool} {"FFT State"=enum."Configure", "Set FFT State?"=FALSE} ("FFT State"), w65) -> (w71:cluster{"FFT State":T2, "Set FFT State?":bool}[])
  n40 = Build Array (concatenate)(w71, w71, w71, w71) -> (w74:cluster{"FFT State":T2, "Set FFT State?":bool}[])
  n41 = Initialize Array(0.0, w57) -> (w79:dbl[])
  n42 = Initialize Array(FALSE, w57) -> (w76:bool[])
  n43 = Build Array (concatenate)(w64, w64, w64, w64) -> (w75:bool[])
  n44 = Array Size(array=w71) -> (size(s)=w70:i32)
  n45 = Build Array (concatenate)(w66, w66, w66, w66) -> (w78:dbl[])
  n46 = Initialize Array(0.0, w57) -> (w60:dbl[])
  n47 = Build Array (concatenate)(w58, w58, w58, w58) -> (w61:dbl[])
  n48 = Build Array (concatenate)(w73, w74) -> (w72:cluster{"FFT State":T2, "Set FFT State?":bool}[])
  n49 = Compound Arithmetic op=ADD(w70, w57, 10 ("value")) -> (w68:i32)
  n50 = Build Array (concatenate)(w79, w78) -> (w56:dbl[])
  n51 = Build Array (concatenate)(w76, w75) -> (w62:bool[])
  n52 = Build Array (concatenate)(w60, w61) -> (w55:dbl[])
  n53 = Replace Array Subset(array=w72, new element=cluster{"FFT State":T2, "Set FFT State?":bool} {"FFT State"=enum."Unload Last FFT", "Set FFT State?"=TRUE} ("FFT State"), index=w68) -> (w63:cluster{"FFT State":T2, "Set FFT State?":bool}[])
  n54 = for {
    N -> [w165]
    tunnel: [w167] -> w93 mode=indexing
    tunnel: [w171] -> w84
    tunnel: w63 -> [w161] mode=indexing
    tunnel: w62 -> [w156] mode=indexing
    tunnel: w56 -> [w155] mode=indexing
    tunnel: w55 -> [w154] mode=indexing
    tunnel: [w153] -> w51
    tunnel: [w152] -> w52
    tunnel: [w140] -> w50
    tunnel: [w139] -> w49
    tunnel: [w135] -> w38
    tunnel: [w134] -> w37
    i -> [w166]
    n55 = Divide(x=w166, y=w165) -> (x/y=w164:dbl)
    n56 = To Fixed-Point(number=w155) -> (fixed-point=w158:fxp<+/-,16,1>)  [unwired: 1 in]
    n57 = To Fixed-Point(number=w154) -> (fixed-point=w157:fxp<+/-,16,1>)  [unwired: 1 in]
    n58 = Multiply(x=w164, y=100.0) -> (x*y=→"Test Progress (%)":dbl)
    n59 = call "FFT Process.vi"("FFT Parameters"="FFT Parameters", "FFT State"=w161, "Input Valid"=w156, "Real Data In"=w158) -> ("Imag Data Out"=w144:fxp<+/-,16,1>, "Real Data Out"=w145:fxp<+/-,16,1>, "FFT Status"=w159:T6)  [unwired: 2 in, 3 out]
    n60 = call "FFT Process.vi"("FFT Parameters"="FFT Parameters", "FFT State"=w161, "Input Valid"=w156, "Real Data In"=w157) -> ("Output Valid"=w141:bool, "Imag Data Out"=w142:fxp<+/-,16,1>, "Real Data Out"=w143:fxp<+/-,16,1>, "FFT Status"=w170:T6)  [unwired: 2 in, 2 out]
    n61 = Unbundle By Name(w170) -> ("FFT Overflow"=w168:bool)
    n62 = Unbundle By Name(w159) -> ("FFT Overflow"=w169:bool)
    n63 = call "Combine Two FFTs computed using DIT.vi"("Real FFT 1"=w145, "Imag FFT 1"=w144, "Real FFT 2"=w143, "Imag FFT 2"=w142, "Input Data Valid"=w141) -> ("Real FFT k"=w138:fxp<+/-,24,3>, "Imag FFT k"=w137:fxp<+/-,24,3>, "Output Valid"=w136:bool)  [unwired: 6 in, 2 out]
    n64 = call "Magnitude Square of Complex Number.vi"("Real"=w138, "Imaginary"=w137, "Input Valid"=w136) -> ("Magnitude^2"=w148:fxp<+,48,14>, "Output Valid"=w149:bool)  [unwired: 11 in]
    n65 = To Fixed-Point "+,32,1"(number=w148) -> (fixed-point=w150:fxp<+,32,1>)  [unwired: 1 in]
    n66 = call <userlib>:"Logarithm10 of Number (U32).vi"("Input Valid"=w149, "Input Number (0.32)"=w150) -> ("Output Valid"=w151:bool, "Logarithm"=w147:fxp<+/-,34,12>)  [unwired: 6 in, 2 out]
    n67 = call <userlib>:"Collect Signal on Datavalid.vi"("Data Valid"=w136, "Input"=w138) -> ("Output"=w135:dbl[])  [unwired: 9 in]
    n68 = call <userlib>:"Collect Signal on Datavalid.vi"("Data Valid"=w141, "Input"=w145) -> ("Output"=w152:dbl[])  [unwired: 9 in]
    n69 = call <userlib>:"Collect Signal on Datavalid.vi"("Data Valid"=w141, "Input"=w144) -> ("Output"=w153:dbl[])  [unwired: 9 in]
    n70 = call <userlib>:"Collect Signal on Datavalid.vi"("Data Valid"=w141, "Input"=w143) -> ("Output"=w140:dbl[])  [unwired: 9 in]
    n71 = call <userlib>:"Collect Signal on Datavalid.vi"("Data Valid"=w141, "Input"=w142) -> ("Output"=w139:dbl[])  [unwired: 9 in]
    n72 = call <userlib>:"Collect Signal on Datavalid.vi"("Data Valid"=w136, "Input"=w137) -> ("Output"=w134:dbl[])  [unwired: 9 in]
    n73 = To Fixed-Point(number=w147) -> (fixed-point=w146:fxp<+/-,16,8>)  [unwired: 1 in]
    n74 = Or(x=w169, y=w168) -> (x .or. y?=w167:bool)
    n75 = call <userlib>:"Collect Signal on Datavalid.vi"("Data Valid"=w151, "Input"=w146) -> ("Output"=w171:dbl[])  [unwired: 9 in]
    "Iterations" <- w165
  }
  n76 = Re/Im To Complex(1:w37, 2:w38) -> (0:w36:cdb[])
  n77 = Or Array Elements(Boolean array=w93) -> (logical OR=→"FFT Overflow?":bool)
  n78 = Array Size(array=w52) -> (size(s)=w53:i32)
  n79 = Re/Im To Complex(1:w51, 2:w52) -> (0:w46:cdb[])
  n80 = Re/Im To Complex(1:w49, 2:w50) -> (0:w48:cdb[])
  n81 = Absolute Value(x=w36) -> (abs(x)=w35:dbl[])
  n82 = mathscript code="k=0:N-1;\nW=exp(-j*pi*k/N);"("N"=w53) -> ("W"=w47:cdb[])  [unwired: 1 in, 1 out]
  n83 = Square(x=w35) -> (x^2=w34:dbl[])
  n84 = Logarithm Base 10(1:w34) -> (0:w33:dbl[])
  n85 = Multiply(x=10, y=w33) -> (x*y=w31:dbl[])
  n86 = Subtract(x=w84, y=w11) -> (x-y=w91:dbl[])
  "Error Signal" <- w91
  n87 = Subtract(x=w31, y=w11) -> (x-y=→"Error 2":dbl[])
  n88 = Multiply(x=w47, y=w48) -> (x*y=w45:cdb[])
  n89 = Add(x=w46, y=w45) -> (x+y=w44:cdb[])
  n90 = Absolute Value(x=w91) -> (abs(x)=w94:dbl[])
  n91 = call-poly <vilib>:"FFT Spectrum (Mag-Phase).vi"("view"=T3 {"dB On (F)"=TRUE, "unwrap phase (F)"=FALSE, "convert to degree (F)"=FALSE}, "time signal"=w91) -> ("magnitude"=w92:cluster{"f0":dbl, "df":dbl, "magnitude":dbl[]})  [unwired: 5 in, 4 out]
  "Error Spectrum" <- w92
  n92 = Absolute Value(x=w44) -> (abs(x)=w43:dbl[])
  n93 = Unbundle By Name(w92) -> ("magnitude"=w97:dbl[])
  n94 = Add Array Elements(numeric array=w94) -> (sum=w88:dbl)
  n95 = Square(x=w43) -> (x^2=w41:dbl[])
  n96 = Logarithm Base 10(1:w41) -> (0:w42:dbl[])
  n97 = Multiply(x=10, y=w42) -> (x*y=w6:dbl[])
  "FFT_FXP_no DIT" <- w6
  n98 = Absolute Value(x=w97) -> (abs(x)=w96:dbl[])
  n99 = Subtract(x=w6, y=w11) -> (x-y=→"Error":dbl[])
  n100 = Less?(x=w88, y=0.001) -> (x < y?=w86:bool)
  n101 = Array Max & Min(array=w96) -> (min value=w90:dbl)  [unwired: 3 out]
  n102 = Greater Or Equal?(x=w90, y=55.0) -> (x >= y?=w85:bool)
  n103 = And(x=w86, y=w85) -> ()  [unwired: 1 out]
